vi "Driver Rev.vi"(8 "error in":errorcluster, 11 "Instrument Handle In":i32) -> (0 "error out":errorcluster, 2 "Driver Rev":string caption="Driver Revision", 3 "Instrument Handle Out":i32)   [LabVIEW 8.6, in "ZTScopeM.lvlib"]
doc: "Query the driver revision."
uses:
  ZTScopeM.lvlib
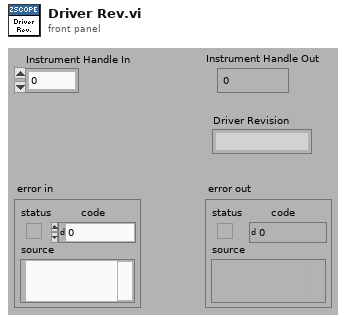
[diagram p1: front panel]
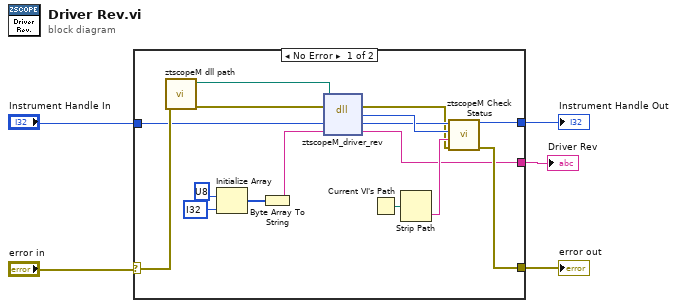
[diagram p0: block diagram]
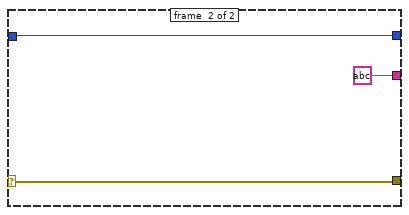
[diagram p2: hidden frame]
diagram:
  n1 = case shown="No Error" "error in" {
    selector: "error in" -> [w10 w24]
    tunnel: [w16 w24] -> w4
    tunnel: [w17 w22] -> w3
    tunnel: [w11 string ? ("driverRev")] -> w2
    tunnel: "Instrument Handle In" -> [w8 w22]
    frame #0 {
      n2 = call "ztscopeM dll path.vi"("error in (no error)"=w10) -> ("error out"=w7:errorcluster, "<instrument>.dll path"=w9:path)  [unwired: 9 in]
      n3 = Initialize Array(u8 ?, i32 ? ("dimension size")) -> (w14:u8[])
      n4 = Byte Array To String(unsigned byte array=w14) -> (string=w12:string)
      n5 = dll-call lib="C:/Program Files (x86)/National Instruments/LabVIEW 2013/instr.lib/ztscopem/ztscopeM.dll" fn="ztscopeM_driver_rev"(path in=w9, error in=w7, "instrumentHandle"=w8, "driverRev"=w12) -> (error out=w6:errorcluster, w21:i32, "instrumentHandle"=w20:i32, "driverRev"=w11:string)  [unwired: 1 in, 1 out]
      n6 = Current VI's Path() -> (path=w19:path)
      n7 = Strip Path(path=w19) -> (name=w18:string)  [unwired: 1 out]
      n8 = call "ztscopeM Check Status.vi"("error in"=w6, "name of VI"=w18, "status (return code)"=w21, "instrument handle in"=w20) -> ("error out"=w16:errorcluster, "instrument handle out"=w17:i32)  [unwired: 2 out]
    }
    frame #1 {
    }
  }
  "Instrument Handle Out" <- w3
  "error out" <- w4
  "Driver Rev" <- w2
